vi "Read Active VI.vi"(8 "error in (no error)":errorcluster, 11 "Panel Actor in":refnum<class "Panel Actor.lvclass">) -> (0 "error out":errorcluster, 2 "Active VI ref":refnum<vi>, 3 "Panel Actor out":refnum<class "Panel Actor.lvclass">)   [LabVIEW 2017, in "MGI-Panel Actor.lvlib" / "Panel Actor.lvclass"]
doc: "Gets the actor VI ref. If no actove VI has been set, this opens a references to the most specific version of Actor Core.\n----\nCopyright: MGI 2018\nAuthor: Derek Trepanier"
uses:
  Panel Actor.lvclass
  Panel Actor.lvclass/Panel Actor.ctl
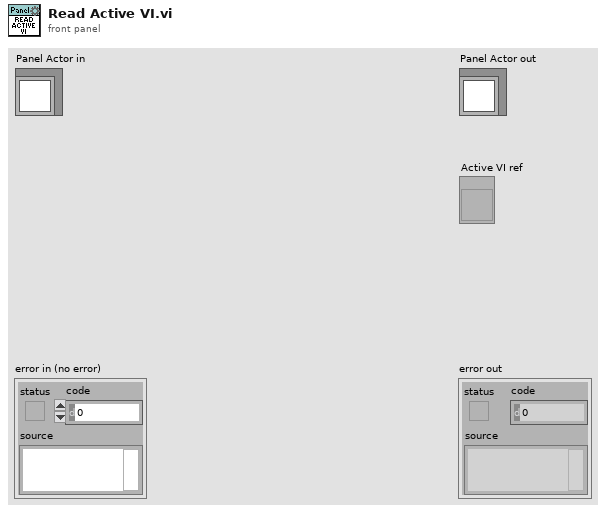
[diagram p1: front panel]
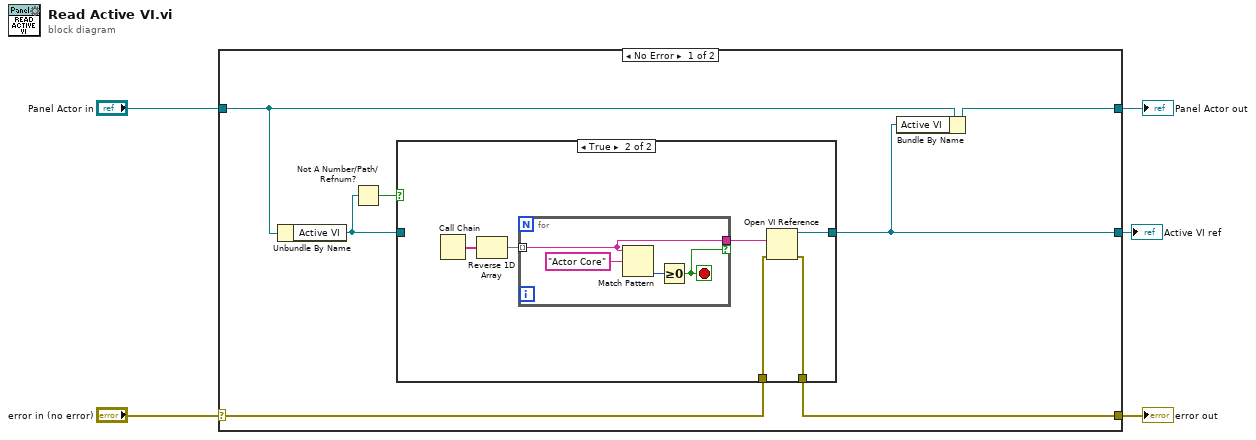
[diagram p0: block diagram]
diagram:
  n1 = case shown="No Error" "error in (no error)" {
    selector: "error in (no error)" -> [w7 w26]
    tunnel: [w6 w26] -> w4
    tunnel: [w9 w25] -> w2
    tunnel: "Panel Actor in" -> [w12 w25]
    tunnel: [w8 _] -> w1
    frame No Error {
      n2 = Unbundle By Name(w12) -> ("Active VI"=w10:refnum<vi>)
      n3 = Not A Number/Path/Refnum?(number/path/refnum=w10) -> (NaN/Path/Refnum?=w11:bool)
      n4 = case shown="True" w11 {
        tunnel: w10 -> [w14 _]
        tunnel: [w14 w17] -> w8
        tunnel: w7 -> [w13 w16]
        tunnel: [w13 w15] -> w6
        frame False {
        }
        frame True {
          n5 = Call Chain() -> (call chain=w20:string[])
          n6 = Reverse 1D Array(array=w20) -> (reversed array=w19:string[])
          n7 = for {
            tunnel: w19 -> [w22] mode=indexing
            tunnel: [w22] -> w18 if=w21
            stop <- w21 stop-if-true
            n8 = Match Pattern(string=w22, regular expression="Actor Core") -> (offset past match=w23:i32)  [unwired: 1 in, 3 out]
            n9 = Greater Or Equal To 0?(x=w23) -> (x >= 0?=w21:bool)
          }
          n10 = Open VI Reference(vi path=w18, error in (no error)=w16) -> (vi reference=w17:refnum<vi>, error out=w15:errorcluster)  [unwired: 4 in]
        }
      }
      n11 = Bundle By Name(cluster=w12, "Active VI"=w8) -> (w9:refnum<class "Panel Actor.lvclass">)
    }
    frame Error {
    }
  }
  "error out" <- w4
  "Panel Actor out" <- w2
  "Active VI ref" <- w1
